vi "Extended.BuildSysexMsgI2CConfig.vi"(8 "error in":errorcluster, 9 "msDelay (Optional)":u8) -> (0 "error out":errorcluster, 1 "ReplyLength":i32=-1, 2 "ReplyFirstByte":T1=224 items=["ANALOG_IO_MESSAGE"=224, "DIGITAL_IO_MESSAGE"=144, "REPORT_ANALOG_PIN"=192, "REPORT_DIGITAL_PORT"=208, "START_SYSEX"=240, "END_SYSEX"=247, "SET_PIN_MODE"=244, "SET_DIGITAL_PIN_VALUE"=245, "PROTOCOL_VERSION"=249, "SYSTEM_RESET"=255, "SYSEX.EXTENDED_ID"=0, "SYSEX.RESERVED_USER_COMMANDs"=1, "SYSEX.ANALOG_MAPPING_QUERY"=105, "SYSEX.ANALOG_MAPPING_RESPONSE"=106, "SYSEX.CAPABILITY_QUERY"=107, "SYSEX.CAPABILITY_RESPONSE"=108, "SYSEX.PIN_STATE_QUERY"=109, "SYSEX.PIN_STATE_RESPONSE"=110, "SYSEX.REPORT_FIRMWARE"=121, "SYSEX.EXTENDED_ANALOG"=111, "SYSEX.STRING_DATA"=113, "SYSEX.REALTIME"=127, "SYSEX.NON_REALTIME"=126, "SYSEX.SAMPLING_INTERVAL"=122], 3 "GetPinStateMessage":u8[](array[numeric]) format="%x")   [LabVIEW 2020, in "FirmataClient.lvlib"]
doc: "Builds a message according to the Firmata Protocol Requirements. \n- https://github.com/firmata/protocol\n- https://github.com/firmata/protocol/blob/master/protocol.md"
uses:
  FirmataClient.lvlib
  controls/FirmataProtocolConstants.ctl
  147f2e90-8315-44ff-bc99-ac74707c4f68.vi
  private/Transform8BitsInArray.vi
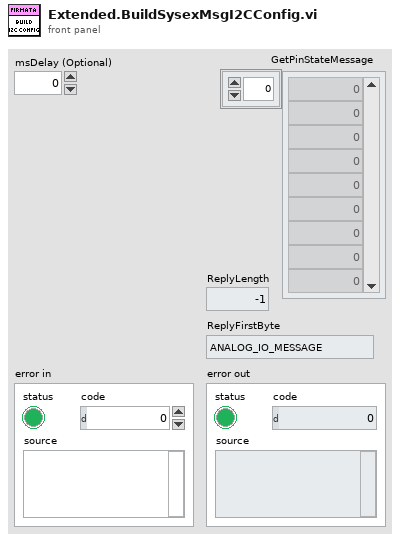
[diagram p1: front panel]
types:
  T1 = typedef "FirmataClient.lvlib/FirmataProtocolConstants.ctl" = u16
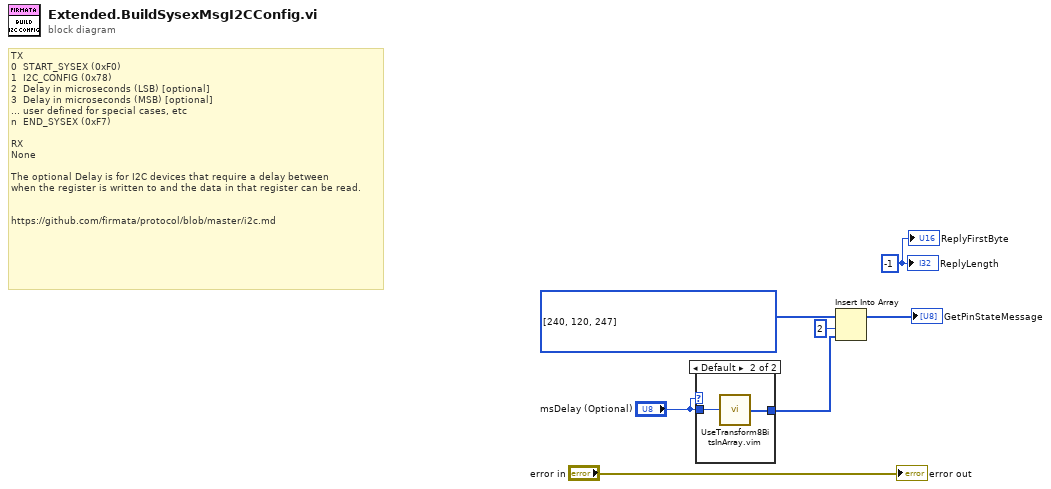
[diagram p0: block diagram]
diagram:
  w6 = -1 ("ReplyLength")
  w4 = T1[] [240, 120, 247] items=["ANALOG_IO_MESSAGE"=224, "DIGITAL_IO_MESSAGE"=144, "REPORT_ANALOG_PIN"=192, "REPORT_DIGITAL_PORT"=208, "START_SYSEX"=240, "END_SYSEX"=247, "SET_PIN_MODE"=244, "SET_DIGITAL_PIN_VALUE"=245, "PROTOCOL_VERSION"=249, "SYSTEM_RESET"=255, "SYSEX.EXTENDED_ID"=0, "SYSEX.RESERVED_USER_COMMANDs"=1, "SYSEX.ANALOG_MAPPING_QUERY"=105, "SYSEX.ANALOG_MAPPING_RESPONSE"=106, "SYSEX.CAPABILITY_QUERY"=107, "SYSEX.CAPABILITY_RESPONSE"=108, "SYSEX.PIN_STATE_QUERY"=109, "SYSEX.PIN_STATE_RESPONSE"=110, "SYSEX.REPORT_FIRMWARE"=121, "SYSEX.EXTENDED_ANALOG"=111, "SYSEX.STRING_DATA"=113, "SYSEX.REALTIME"=127, "SYSEX.NON_REALTIME"=126, "SYSEX.SAMPLING_INTERVAL"=122, "FEATURES.SYSEX.I2C_READ_WRITE"=118, "FEATURES.SYSEX.I2C_REPLY"=119, "FEATURES.SYSEX.I2C_CONFIG"=120]
  # "TX\n0  START_SYSEX (0xF0)\n1  I2C_CONFIG (0x78)\n2  Delay in microseconds (LSB) [optional]\n3  Delay in microseconds (MSB) [optional]\n... user defined for special cases, etc\nn  END_SYSEX (0xF7)\n\nRX\nNone\n\nThe optional Delay is for I2C devices that require a delay between \nwhen the register is written to and the data in that register can be read.\n\n\nhttps://github.com/firmata/protocol/blob/master/i2c.md"
  n1 = case shown="Default" "msDelay (Optional)" {
    tunnel: "msDelay (Optional)" -> [_ w9]
    tunnel: [_ w8] -> w2
    frame ..0 {
    }
    frame Default {
      n2 = call "UseTransform8BitsInArray.vim"("Byte In"=w9) -> ("Byte Out"=w8:u32[])
    }
  }
  n3 = Insert Into Array(array=w4, index=2, new element=w2) -> (→"GetPinStateMessage":T1[])
  "error out" <- "error in"
  "ReplyFirstByte" <- w6
  "ReplyLength" <- w6
